vi "ManageFiles.vi"(0 "VISA IN":refnum<visa-resource-name>, 3 "FileName":string, 4 "TgtFileName":string, 5 "error in":errorcluster, 7 "Cmd":string(combo), 9 "FileType":string(combo)="CSA") -> (14 "VISA Out":refnum<visa-resource-name>, 19 "error out":errorcluster)   [LabVIEW 2018, in "PNA-X.lvlib"]
uses:
  PNA-X.lvlib
panel:
  in  "Type":string(combo)
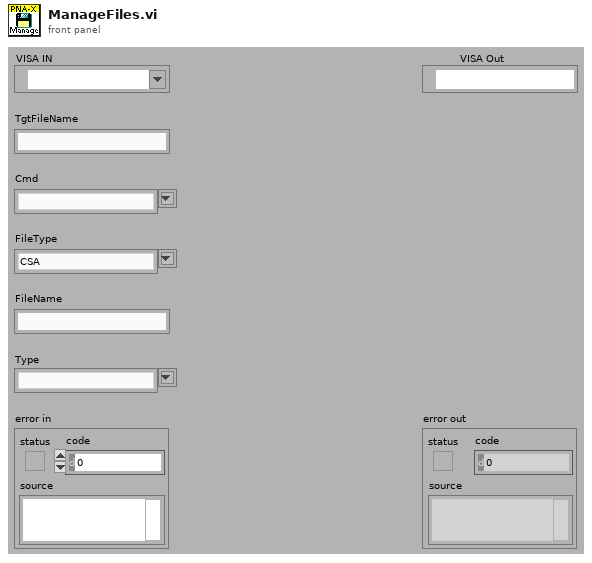
[diagram p1: front panel]
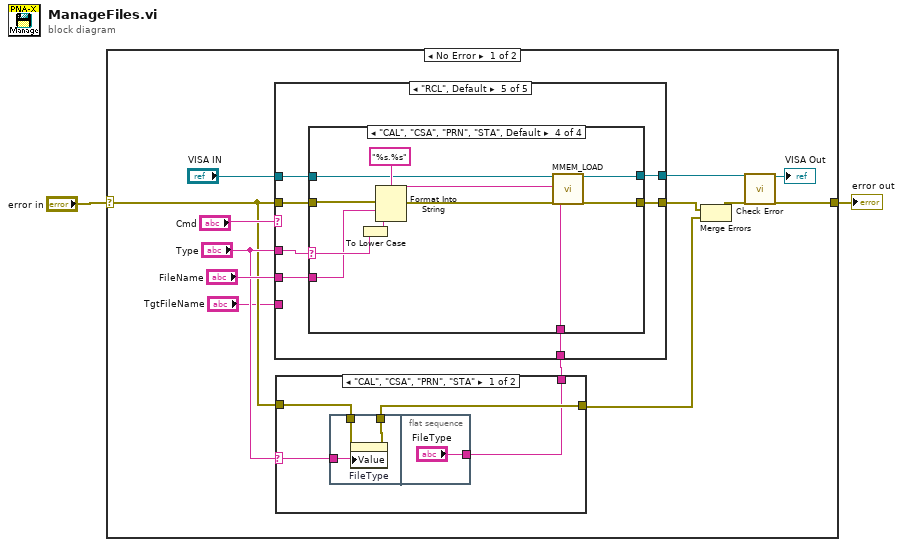
[diagram p0: block diagram]
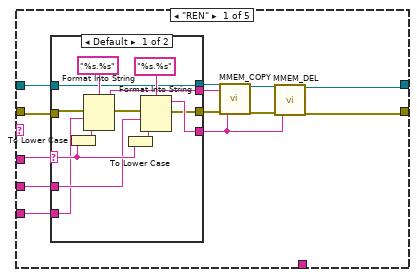
[diagram p3: hidden frame]
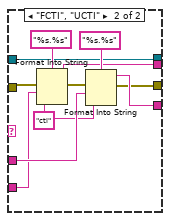
[diagram p4: hidden frame]
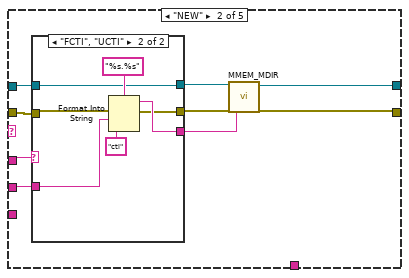
[diagram p5: hidden frame]
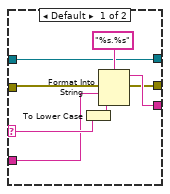
[diagram p6: hidden frame]
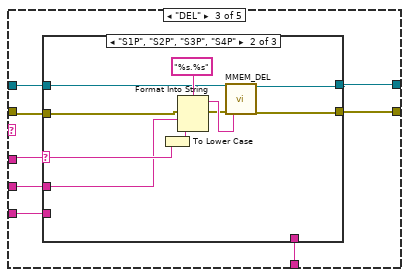
[diagram p7: hidden frame]
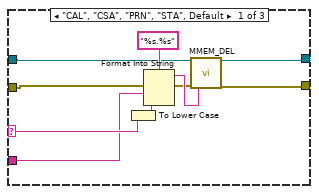
[diagram p8: hidden frame]
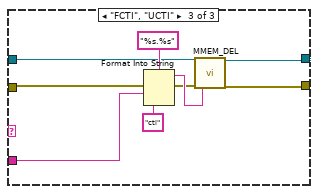
[diagram p9: hidden frame]
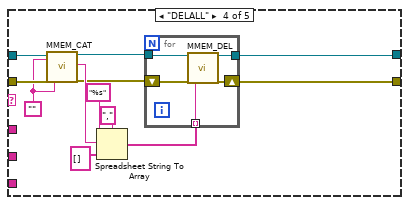
[diagram p10: hidden frame]
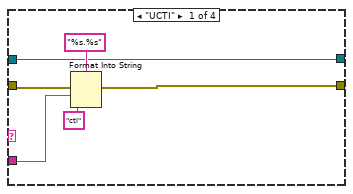
[diagram p11: hidden frame]
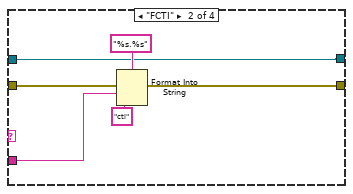
[diagram p12: hidden frame]
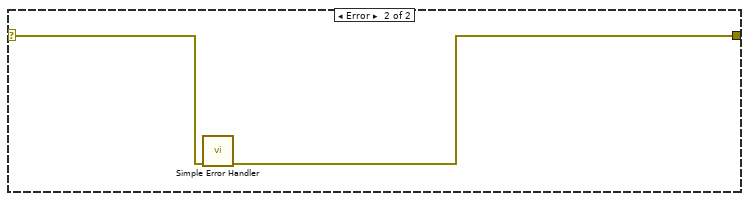
[diagram p14: hidden frame]
diagram:
  n1 = case shown="No Error" "error in" {
    selector: "error in" -> [w10 w173]
    tunnel: [w15 w172] -> w2
    frame No Error {
      n2 = case shown="\"CAL\", \"CSA\", \"PRN\", \"STA\"" "Type" {
        selector: "Type" -> [w19 _]
        tunnel: w10 -> [w18 w24]
        tunnel: [w17 w24] -> w5
        tunnel: [w16 _] -> w9
        frame "CAL", "CSA", "PRN", "STA" {
          n3 = flat-sequence {
            tunnel: w19 -> [w22]
            tunnel: w18 -> [w21]
            tunnel: [w20] -> w17
            tunnel: ["FileType"] -> w16
            frame #0 {
              n4 = property on="FileType" class="CmbBox"(error in=w21, "Value"=w22) -> (error out=w20:errorcluster)  [unwired: 1 in, 1 out]
            }
            frame #1 {
            }
          }
        }
        frame Default {
        }
      }
      n5 = case shown="\"RCL\", Default" "Cmd" {
        tunnel: [w25 w63 w93 w124 w145] -> w6
        tunnel: w10 -> [w37 w70 w92 w134 w146]
        tunnel: "Type" -> [w34 w68 w88 _ w144]
        tunnel: "FileName" -> [w35 w67 w89 _ w142]
        tunnel: w9 -> [_ _ w91 _ w141]
        tunnel: "VISA IN" -> [w36 w69 w90 w133 w143]
        tunnel: "TgtFileName" -> [w33 _ w87 _ _]
        tunnel: [w26 w62 w86 w123 w140] -> w3
        frame "REN" {
          n6 = case shown="Default" w34 {
            selector: w34 -> [w45 _]
            tunnel: [w38 w53] -> w30
            tunnel: [w39 w51] -> w28
            tunnel: w37 -> [w47 w60]
            tunnel: w36 -> [w39 w51]
            tunnel: w35 -> [w44 w58]
            tunnel: w33 -> [w42 w56]
            tunnel: [w41 w54] -> w29
            tunnel: [w40 w52] -> w27
            frame Default {
              n7 = To Lower Case(string=w45) -> (all lower case string=w49:string)
              n8 = Format Into String(format string="%s.%s", error in=w47, w42, w49) -> (resulting string=w40:string, error out=w46:errorcluster)  [unwired: 1 in]
              n9 = To Lower Case(string=w45) -> (all lower case string=w48:string)
              n10 = Format Into String(format string="%s.%s", error in=w46, w44, w48) -> (resulting string=w41:string, error out=w38:errorcluster)  [unwired: 1 in]
            }
            frame "FCTI", "UCTI" {
              w55 = "cti" ("input 2")
              n11 = Format Into String(format string="%s.%s", error in=w60, w56, w55) -> (resulting string=w52:string, error out=w59:errorcluster)  [unwired: 1 in]
              n12 = Format Into String(format string="%s.%s", error in=w59, w58, w55) -> (resulting string=w54:string, error out=w53:errorcluster)  [unwired: 1 in]
            }
          }
          n13 = call "MMEM_COPY.vi"("VISA IN"=w28, "Tgt"=w27, "error in"=w30, "Src"=w29) -> ("VISA Out"=w31:refnum<visa-resource-name>, "error out"=w32:errorcluster)  [unwired: 14 in]
          n14 = call "MMEM_DEL.vi"("VISA IN"=w31, "error in"=w32, "File"=w29) -> ("VISA Out"=w26:refnum<visa-resource-name>, "error out"=w25:errorcluster)  [unwired: 15 in]
        }
        frame "NEW" {
          n15 = case shown="\"FCTI\", \"UCTI\"" w68 {
            selector: w68 -> [w77 _]
            tunnel: [w72 w81] -> w65
            tunnel: [w73 w80] -> w66
            tunnel: w70 -> [w71 w79]
            tunnel: w69 -> [w73 w80]
            tunnel: w67 -> [w76 w85]
            tunnel: [w74 w82] -> w64
            frame Default {
              n16 = To Lower Case(string=w77) -> (all lower case string=w78:string)
              n17 = Format Into String(format string="%s.%s", error in=w71, w76, w78) -> (resulting string=w74:string, error out=w72:errorcluster)  [unwired: 1 in]
            }
            frame "FCTI", "UCTI" {
              n18 = Format Into String(format string="%s.%s", error in=w79, w85, "cti" ("input 2")) -> (resulting string=w82:string, error out=w81:errorcluster)  [unwired: 1 in]
            }
          }
          n19 = call "MMEM_MDIR.vi"("VISA IN"=w66, "error in"=w65, "Folder"=w64) -> ("VISA Out"=w62:refnum<visa-resource-name>, "error out"=w63:errorcluster)  [unwired: 15 in]
        }
        frame "DEL" {
          n20 = case shown="\"S1P\", \"S2P\", \"S3P\", \"S4P\"" w88 {
            selector: w88 -> [w102 w112 _]
            tunnel: [w99 w109 w120] -> w93
            tunnel: [w98 w108 w119] -> w86
            tunnel: w92 -> [w96 w106 w115]
            tunnel: w91 -> [_ _ _]
            tunnel: w90 -> [w95 w104 w116]
            tunnel: w89 -> [w101 w111 w122]
            tunnel: w87 -> [_ _ _]
            frame "CAL", "CSA", "PRN", "STA", Default {
              n21 = To Lower Case(string=w102) -> (all lower case string=w103:string)
              n22 = Format Into String(format string="%s.%s", error in=w96, w101, w103) -> (resulting string=w97:string, error out=w94:errorcluster)  [unwired: 1 in]
              n23 = call "MMEM_DEL.vi"("VISA IN"=w95, "error in"=w94, "File"=w97) -> ("VISA Out"=w98:refnum<visa-resource-name>, "error out"=w99:errorcluster)  [unwired: 15 in]
            }
            frame "S1P", "S2P", "S3P", "S4P" {
              n24 = To Lower Case(string=w112) -> (all lower case string=w113:string)
              n25 = Format Into String(format string="%s.%s", error in=w106, w111, w113) -> (resulting string=w107:string, error out=w105:errorcluster)  [unwired: 1 in]
              n26 = call "MMEM_DEL.vi"("VISA IN"=w104, "error in"=w105, "File"=w107) -> ("VISA Out"=w108:refnum<visa-resource-name>, "error out"=w109:errorcluster)  [unwired: 15 in]
            }
            frame "FCTI", "UCTI" {
              n27 = Format Into String(format string="%s.%s", error in=w115, w122, "cti" ("input 2")) -> (resulting string=w118:string, error out=w117:errorcluster)  [unwired: 1 in]
              n28 = call "MMEM_DEL.vi"("VISA IN"=w116, "error in"=w117, "File"=w118) -> ("VISA Out"=w119:refnum<visa-resource-name>, "error out"=w120:errorcluster)  [unwired: 15 in]
            }
          }
        }
        frame "DELALL" {
          w132 = ""
          n29 = call "MMEM_CAT.vi"("VISA IN"=w133, "Folder"=w132, "error in"=w134, "Types"=w132) -> ("VISA Out"=w125:refnum<visa-resource-name>, "Data"=w131:string, "error out"=w126:errorcluster)  [unwired: 13 in]
          n30 = Spreadsheet String To Array(delimiter (Tab)=",", format string="%s", spreadsheet string=w131, array type (2D Dbl)=string[] []) -> (array=w128:string[])
          n31 = for {
            tunnel: w128 -> [w137] mode=indexing
            tunnel: w125 -> [w138]
            shift-right: [w136] -> w124
            shift-left: w126 -> [w139]
            tunnel: [w135] -> w123
            n32 = call "MMEM_DEL.vi"("VISA IN"=w138, "error in"=w139, "File"=w137) -> ("VISA Out"=w135:refnum<visa-resource-name>, "error out"=w136:errorcluster)  [unwired: 15 in]
          }
        }
        frame "RCL", Default {
          n33 = case shown="\"CAL\", \"CSA\", \"PRN\", \"STA\", Default" w144 {
            selector: w144 -> [_ _ _ w168]
            tunnel: [w149 w155 w160 w171] -> w145
            tunnel: [w147 w154 w159 w170] -> w140
            tunnel: w146 -> [w150 w156 w160 w166]
            tunnel: w143 -> [w147 w154 w159 w164]
            tunnel: w142 -> [w148 w153 _ w163]
            tunnel: w141 -> [_ _ _ w161]
            frame "UCTI" {
              n34 = Format Into String(format string="%s.%s", error in=w150, w148, "cti" ("input 2")) -> (error out=w149:errorcluster)  [unwired: 1 in, 1 out]
            }
            frame "FCTI" {
              n35 = Format Into String(format string="%s.%s", error in=w156, w153, "cti" ("input 2")) -> (error out=w155:errorcluster)  [unwired: 1 in, 1 out]
            }
            frame "S1P", "S2P", "S3P", "S4P" {
            }
            frame "CAL", "CSA", "PRN", "STA", Default {
              n36 = To Lower Case(string=w168) -> (all lower case string=w167:string)
              n37 = Format Into String(format string="%s.%s", error in=w166, w163, w167) -> (resulting string=w165:string, error out=w162:errorcluster)  [unwired: 1 in]
              n38 = call "MMEM_LOAD.vi"("VISA IN"=w164, "FileName"=w165, "error in"=w162, "FileType"=w161) -> ("VISA Out"=w170:refnum<visa-resource-name>, "error out"=w171:errorcluster)  [unwired: 14 in]
            }
          }
        }
      }
      n39 = Merge Errors(w6, w5) -> (w7:errorcluster)
      n40 = call "Check Error.vi"("VISA Resource Name"=w3, "error in (no error)"=w7) -> ("dup VISA session"=→"VISA Out":refnum<visa-resource-name>, "error out"=w15:errorcluster)  [unwired: 16 in]
    }
    frame Error {
      n41 = call <vilib>:"Simple Error Handler.vi"("error in (no error)"=w173) -> ("error out"=w172:errorcluster)  [unwired: 4 in, 4 out]
    }
  }
  "error out" <- w2
